vi "host.vi"() -> ()   [LabVIEW 2020]
uses:
  <vilib>/FPGAPlugInAG/cRIO-9035/niLvFpga_Open_cRIO-9035.vi
  <vilib>/rvi/interface/common/dynamic/niFpgaDynamicAddResources.vi
  <vilib>/Utility/error.llb/Error Cluster From Error Code.vi
  <vilib>/rvi/interface/common/niFpgaWaitOnOcc.vi
  <vilib>/rvi/errors/niLvFpgaAdjustHostInterfaceError.vi
  <vilib>/FPGAPlugInAG/Dynamic/niLvFpga_Run_Dynamic.vi
  <vilib>/FPGAPlugInAG/Dynamic/niLvFpga_Close_Dynamic.vi
  <vilib>/rvi/interface/nirviOpenFPGA/nirviOpenFPGA.xnode
  FPGA Bitfiles/fftfpgaapplicati_FPGATarget_FFT2_KeSgG5ORnEI.lvbitx
  FFT.vi
  <vilib>/rvi/interface/nirviMethod/nirviMethod.xnode
  <vilib>/rvi/interface/nirviCloseFPGA/nirviCloseFPGA.xnode
  <vilib>/rvi/errors/niLvFpgaMergeErrorWithErrorCode.vi
  <vilib>/FPGAPlugInAG/Dynamic/niLvFpga_ReadFifo_Dynamic.vi
  <vilib>/Analysis/NI_AALPro.lvlib
  <vilib>/FPGAPlugInAG/Dynamic/niLvFpga_ConfigureFifo_Dynamic.vi
  <vilib>/FPGAPlugInAG/Dynamic/niLvFpga_StartFifo_Dynamic.vi
  <vilib>/FPGAPlugInAG/Dynamic/niLvFpga_WriteFifo_Dynamic.vi
panel:
  out "Actual Depth":u32
  out "img 1":u32
  out "real 1":u32
  out "host to target":u32
  out "signal_target_to_host_fixed size(s)":i32
  out "target to host 1":u32
  out "signal target to host":dbl[][](graph)
  out "signal_target_to_host_fixed":fxp<+/-,24,7>[](array[numeric])
  out "Array 2":fxp<+/-,24,7>[](array[numeric])
  out "img array size":i32
  out "real array size":i32
  out "img Fixed":fxp<+/-,32,21>[](array[numeric])
  out "real Fixed":fxp<+/-,32,21>[](array[numeric])
  out "detrend acc":dbl[](graph)
  out "acc":dbl[](graph)
  out "samples":i32
  out "Waveform Graph":dbl[][](graph)
  out "input signal":T1(graph)
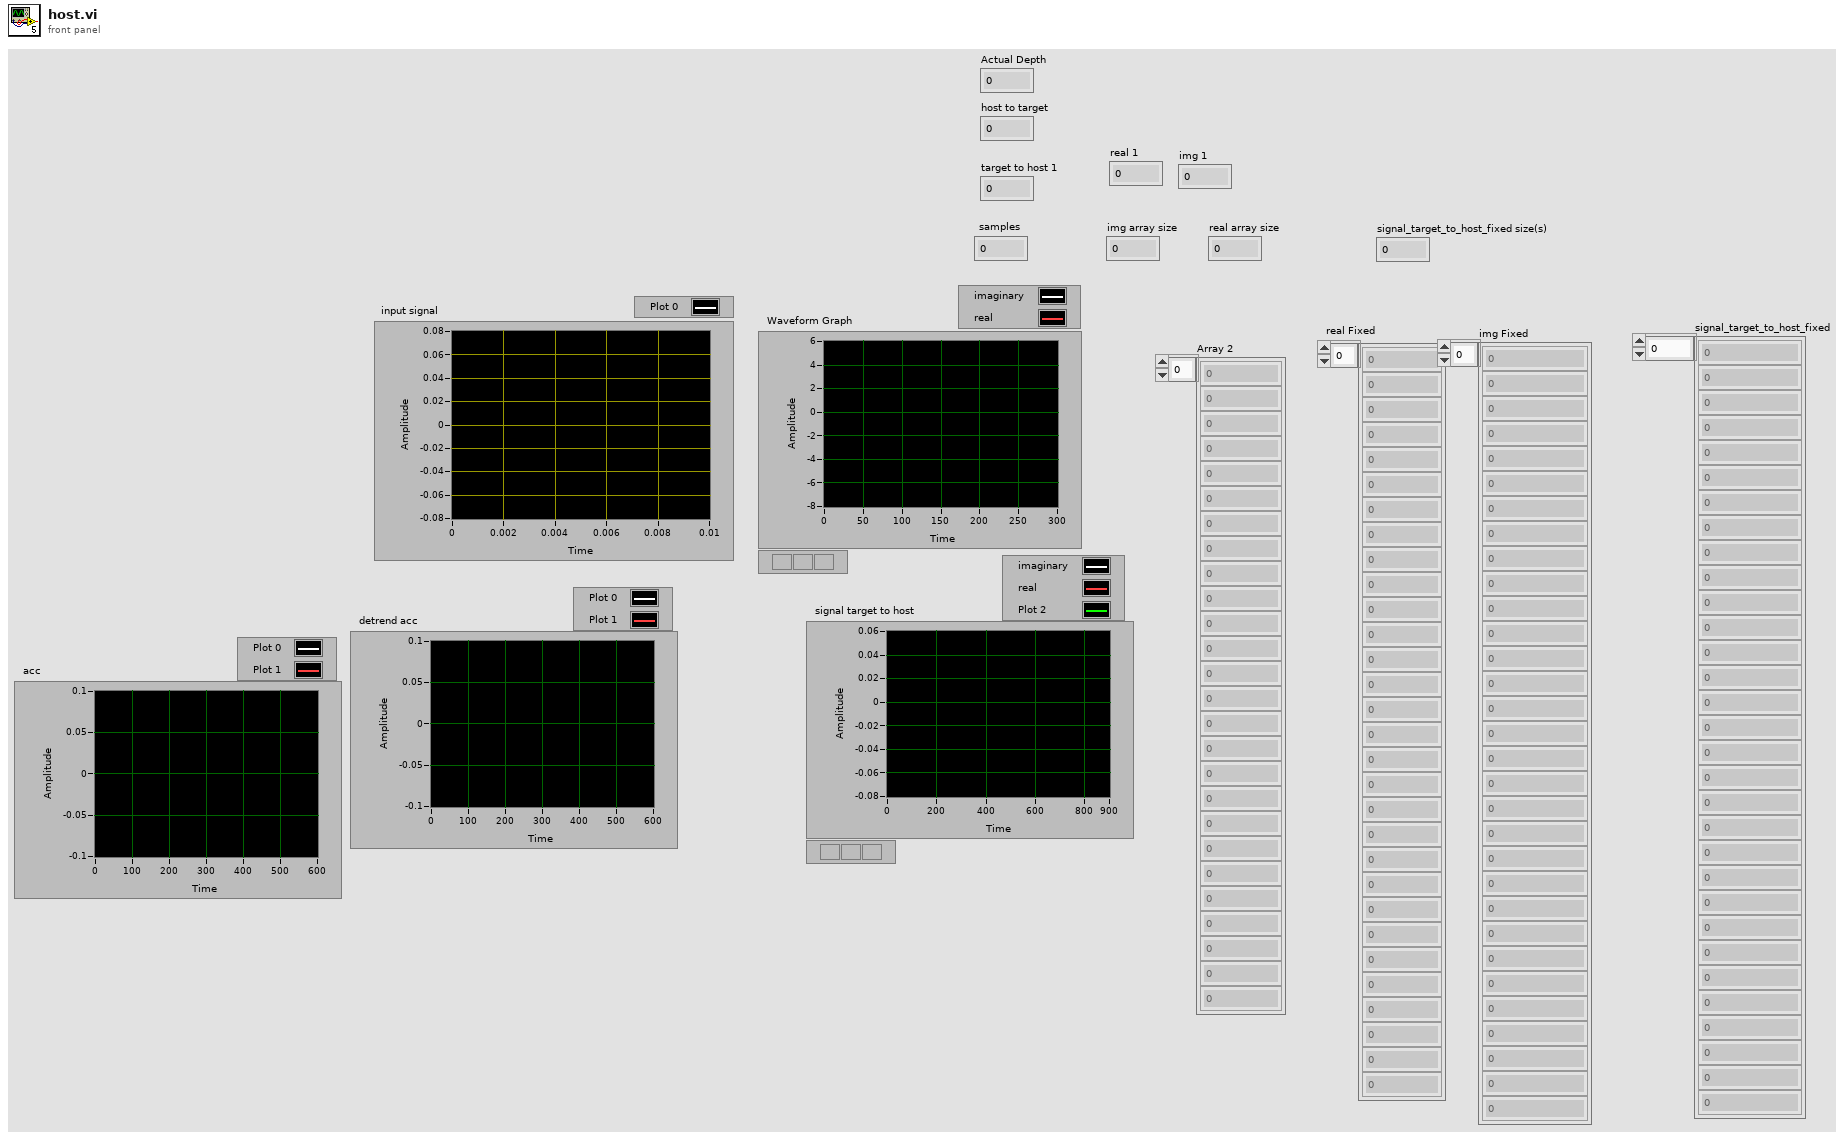
[diagram p1: front panel]
types:
  T1 = cluster{"array type (2D Dbl)":dbl[], "array type (2D Dbl)":dbl[]}
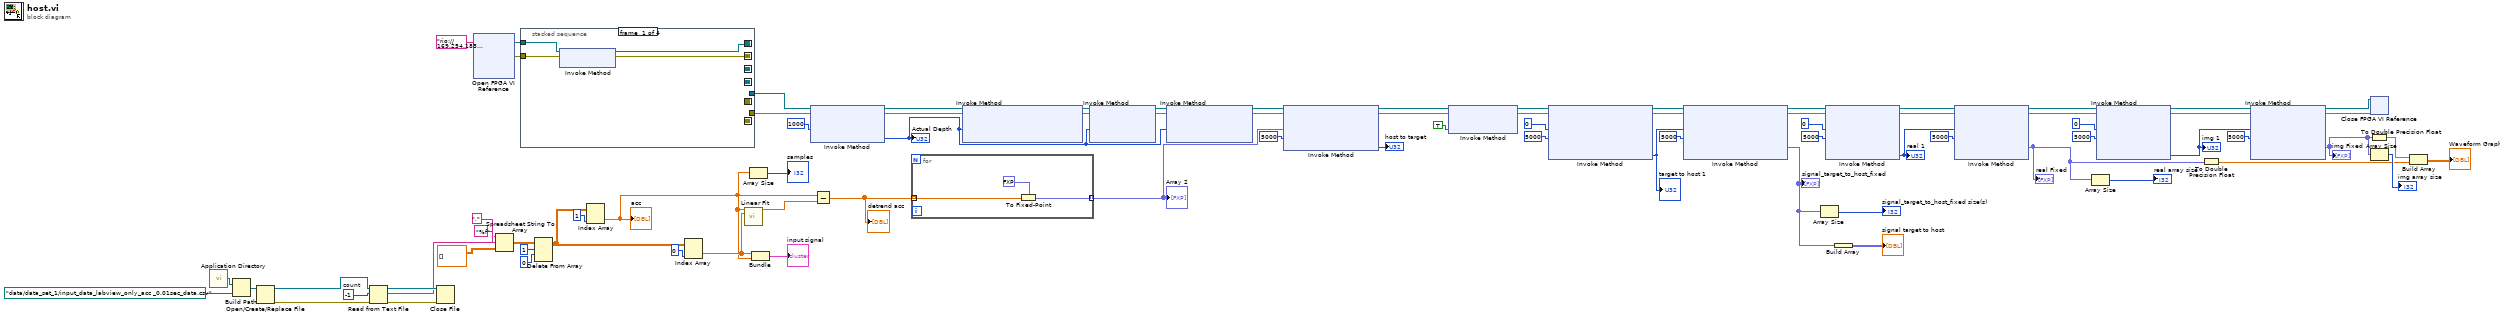
[diagram p0: block diagram]
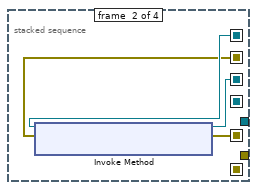
[diagram p2: hidden frame]
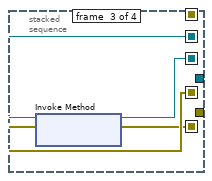
[diagram p3: hidden frame]
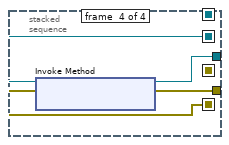
[diagram p4: hidden frame]
diagram:
  w72 = -1  # count
  n1 = call <vilib>:"Application Directory.vi"() -> ("Application Directory"=w76:path)
  n2 = Build Path(base path=w76, name or relative path=path "data/data_set_1/input_data_labview_only_acc _0.01sec_data.csv" ("default name")) -> (appended path=w75:path)
  n3 = Open/Create/Replace File(file path (use dialog)=w75) -> (refnum out=w80:refnum<file>, error out=w81:errorcluster)  [unwired: 5 in, 1 out]
  n4 = Read from Text File(file (use dialog)=w80, count=w72, error in=w81) -> (refnum out=w79:refnum<file>, text=w77:string, error out=w78:errorcluster)  [unwired: 1 in, 1 out]
  n5 = Close File(refnum=w79, error in=w78) -> ()  [unwired: 2 out]
  n6 = xnode "Open FPGA VI Reference"("resource name"=tag "rio://169.254.183.73/RIO0") -> ("FPGA VI Reference Out"=w14:refnum<k20>, "error out"=w13:errorcluster)  [unwired: 1 in]
  n7 = Spreadsheet String To Array(delimiter (Tab)=",", format string="%f", spreadsheet string=w77, array type (2D Dbl)=dbl[][] []) -> (array=w69:dbl[][])
  n8 = stacked-sequence {
    seq-local: [w83 _ _ _] -> [_ w89 _ _]
    seq-local: [w82 _ _ _] -> [_ w88 _ _]
    seq-local: [_ w87 _ _] -> [_ _ w93 _]
    seq-local: [_ w86 _ _] -> [_ _ w92 _]
    seq-local: [_ _ w91 _] -> [_ _ _ w97]
    seq-local: [_ _ w90 _] -> [_ _ _ w96]
    tunnel: w14 -> [w85 _ _ _]
    tunnel: w13 -> [w84 _ _ _]
    tunnel: [_ _ _ w95] -> w12
    tunnel: [_ _ _ w94] -> w11
    frame #0 {
      n9 = xnode "Invoke Method"("FPGA VI Reference In"=w85, "error in"=w84) -> ("FPGA VI Reference Out"=w83:refnum<k20>, "error out"=w82:errorcluster)
    }
    frame #1 {
      n10 = xnode "Invoke Method"("FPGA VI Reference In"=w89, "error in"=w88) -> ("FPGA VI Reference Out"=w87:refnum<k20>, "error out"=w86:errorcluster)
    }
    frame #2 {
      n11 = xnode "Invoke Method"("FPGA VI Reference In"=w93, "error in"=w92) -> ("FPGA VI Reference Out"=w91:refnum<k20>, "error out"=w90:errorcluster)
    }
    frame #3 {
      n12 = xnode "Invoke Method"("FPGA VI Reference In"=w97, "error in"=w96) -> ("FPGA VI Reference Out"=w95:refnum<k20>, "error out"=w94:errorcluster)
    }
  }
  n13 = Delete From Array(array=w69, length=1, index (row)=0) -> (array with subset deleted=w64:dbl[][])  [unwired: 1 in, 1 out]
  n14 = Index Array(array=w64, index (col)=1 ("disabled index (col)")) -> (element=w39:dbl[])  [unwired: 1 in]
  "acc" <- w39
  n15 = Index Array(array=w64, index (col)=0 ("disabled index (col)")) -> (element=w41:dbl[])  [unwired: 1 in]
  n16 = call <vilib>:"Linear Fit.vi"("Y"=w39, "X"=w41) -> ("Best Linear Fit"=w40:dbl[])  [unwired: 9 in, 4 out]
  n17 = Array Size(array=w39) -> (size(s)=→"samples":i32)
  n18 = Bundle("array type (2D Dbl)"=w41, "array type (2D Dbl)"=w39) -> (→"input signal":T1)  [unwired: 1 in]
  n19 = xnode "Invoke Method"("FPGA VI Reference In"=w12, "error in"=w11, "Requested Depth"=u32 1000) -> ("FPGA VI Reference Out"=w10:refnum<k20>, "error out"=w9:errorcluster, "Actual Depth"=w1:u32)
  "Actual Depth" <- w1
  n20 = Subtract(x=w39, y=w40) -> (x-y=w35:dbl[])
  "detrend acc" <- w35
  n21 = for {
    tunnel: [w99] -> w34 mode=indexing
    tunnel: w35 -> [w98] mode=indexing
    n22 = To Fixed-Point(fixed-point type=fxp<+/-,24,7> 0.0 ("f"), number=w98) -> (fixed-point=w99:fxp<+/-,24,7>)
  }
  "Array 2" <- w34
  n23 = xnode "Invoke Method"("FPGA VI Reference In"=w10, "error in"=w9, "Requested Depth"=w1) -> ("FPGA VI Reference Out"=w8:refnum<k20>, "error out"=w7:errorcluster)  [unwired: 1 out]
  n24 = xnode "Invoke Method"("FPGA VI Reference In"=w8, "error in"=w7, "Requested Depth"=w1) -> ("FPGA VI Reference Out"=w6:refnum<k20>, "error out"=w5:errorcluster)  [unwired: 1 out]
  n25 = xnode "Invoke Method"("FPGA VI Reference In"=w6, "error in"=w5, "Requested Depth"=w1) -> ("FPGA VI Reference Out"=w4:refnum<k20>, "error out"=w3:errorcluster)  [unwired: 1 out]
  n26 = xnode "Invoke Method"("FPGA VI Reference In"=w4, "error in"=w3, "Data"=w34, "Timeout (ms)"=5000) -> ("FPGA VI Reference Out"=w61:refnum<k20>, "error out"=w60:errorcluster, "Empty Elements Remaining"=→"host to target":u32)
  n27 = xnode "Invoke Method"("FPGA VI Reference In"=w61, "error in"=w60, "Wait Until Done (F)"=TRUE) -> ("FPGA VI Reference Out"=w25:refnum<k20>, "error out"=w24:errorcluster)
  n28 = xnode "Invoke Method"("FPGA VI Reference In"=w25, "error in"=w24, "Number of Elements"=u32 0, "Timeout (ms)"=5000) -> ("FPGA VI Reference Out"=w33:refnum<k20>, "error out"=w32:errorcluster, "Elements Remaining"=w31:u32)  [unwired: 1 out]
  "target to host 1" <- w31
  n29 = xnode "Invoke Method"("FPGA VI Reference In"=w33, "error in"=w32, "Number of Elements"=w31, "Timeout (ms)"=5000) -> ("FPGA VI Reference Out"=w23:refnum<k20>, "error out"=w22:errorcluster, "Data"=w27:fxp<+/-,24,7>[])  [unwired: 1 out]
  "signal_target_to_host_fixed" <- w27
  n30 = Array Size(array=w27) -> (size(s)=→"signal_target_to_host_fixed size(s)":i32)
  n31 = xnode "Invoke Method"("FPGA VI Reference In"=w23, "error in"=w22, "Number of Elements"=u32 0, "Timeout (ms)"=5000) -> ("FPGA VI Reference Out"=w59:refnum<k20>, "error out"=w58:errorcluster, "Elements Remaining"=w52:u32)  [unwired: 1 out]
  "real 1" <- w52
  n32 = Build Array(w27) -> (→"signal target to host":fxp<+/-,24,7>[][])
  n33 = xnode "Invoke Method"("FPGA VI Reference In"=w59, "error in"=w58, "Number of Elements"=w52, "Timeout (ms)"=5000) -> ("FPGA VI Reference Out"=w55:refnum<k20>, "error out"=w54:errorcluster, "Data"=w36:fxp<+/-,32,15>[])  [unwired: 1 out]
  "real Fixed" <- w36
  n34 = Array Size(array=w36) -> (size(s)=→"real array size":i32)
  n35 = xnode "Invoke Method"("FPGA VI Reference In"=w55, "error in"=w54, "Number of Elements"=u32 0, "Timeout (ms)"=5000) -> ("FPGA VI Reference Out"=w57:refnum<k20>, "error out"=w56:errorcluster, "Elements Remaining"=w50:u32)  [unwired: 1 out]
  "img 1" <- w50
  n36 = To Double Precision Float(number=w36) -> (double precision float=w19:dbl[])
  n37 = xnode "Invoke Method"("FPGA VI Reference In"=w57, "error in"=w56, "Number of Elements"=w50, "Timeout (ms)"=5000) -> ("FPGA VI Reference Out"=w20:refnum<k20>, "error out"=w16:errorcluster, "Data"=w18:fxp<+/-,32,15>[])  [unwired: 1 out]
  "img Fixed" <- w18
  n38 = xnode "Close FPGA VI Reference"("FPGA VI Reference In"=w20, "error in"=w16) -> ()  [unwired: 1 out]
  n39 = To Double Precision Float(number=w18) -> (double precision float=w17:dbl[])
  n40 = Array Size(array=w18) -> (size(s)=→"img array size":i32)
  n41 = Build Array(w17, w19) -> (→"Waveform Graph":dbl[][])
